vi "Generate Failure Nodes.vi"(10 "Result":T1, 11 "XML Report in":refnum<class "XML Report.lvclass">) -> (3 "XML Report out":refnum<class "XML Report.lvclass">)   [LabVIEW 2020, in "Reports.lvlib" / "XML Report.lvclass"]
uses:
  XML Report.lvclass
  Core/Result/Result.ctl
  Core/Result/Status.ctl
  Core/Result/Type.ctl
  XML Report.lvclass/XML Report.ctl
  <vilib>/Utility/miscctls.llb/LVMapReplaceAction.ctl
  <resource>/objmgr/DOMUserDefRef.rc
  Framework/Utilities/Utilities.lvlib
  Core/Result/Result.lvlib
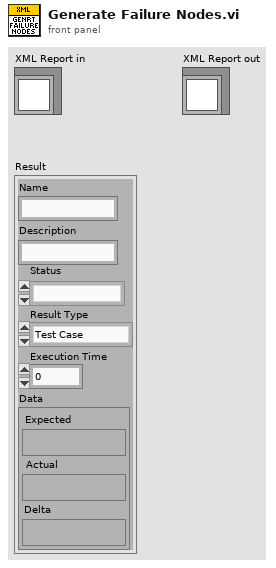
[diagram p1: front panel]
types:
  T1 = typedef "Result.lvlib/Result.ctl" = cluster{"Name":string, "Description":string, "Status":T2, "Result Type":T3, "Execution Time":dbl, "Data":cluster{"Expected":variant, "Actual":variant, "Delta":variant}}
  T2 = typedef "Result.lvlib/Status.ctl" = enum16{"", "Passed", "Failed", "Error", "Skipped", "Setup Error", "Broken", "Teardown Error"}
  T3 = typedef "Result.lvlib/Type.ctl" = enum16{"Test Case", "Test Suite", "Test Run", "Pass", "Fail", "Skip", "Pass if", "Fail if", "Pass if Error", "Fail if Error", "Pass if Equal", "Fail if Equal"}
  T4 = typedef "LVMapReplaceAction.ctl" = enum32{"Modify Entry only if found", "Add or Modify Entry", "Delete Entry"}
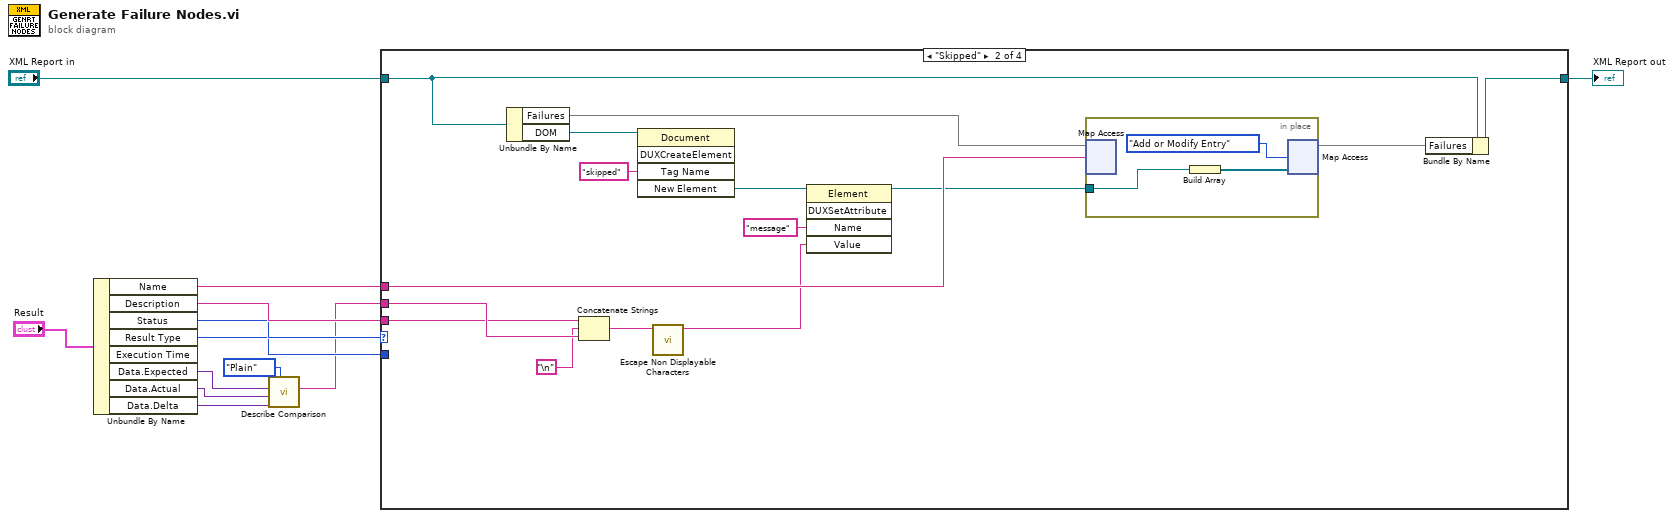
[diagram p0: block diagram]
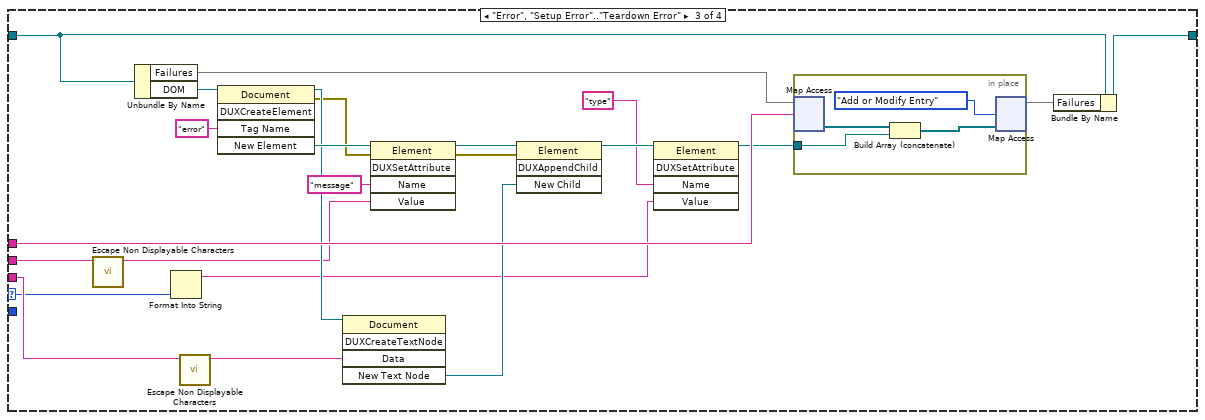
[diagram p3: hidden frame]
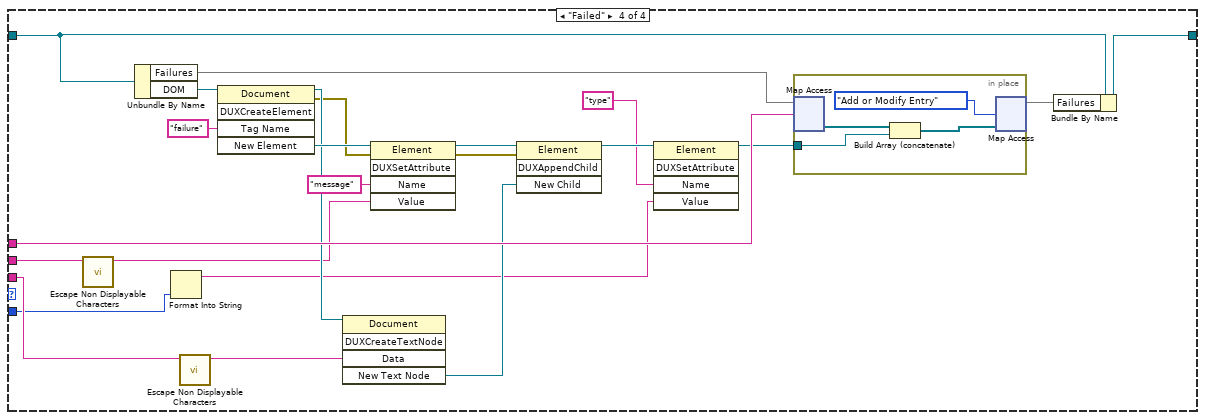
[diagram p4: hidden frame]
diagram:
  n1 = Unbundle By Name("Result") -> ("Name"=w9:string, "Description"=w8:string, "Status"=w7:T2, "Result Type"=w6:T3, "Data.Expected"=w5:variant, "Data.Actual"=w4:variant, "Data.Delta"=w3:variant)  [unwired: 1 out]
  n2 = call "Describe Comparison.vi"("Delta"=w3, "Style"=enum16{"Diff", "Plain"}."Plain", "Actual"=w4, "Expected"=w5) -> ("Description"=w2:string)  [unwired: 7 in]
  n3 = case shown="\"Skipped\"" w7 {
    selector: w7 -> [_ _ w36 _]
    tunnel: [w13 w28 w54 w81] -> w11
    tunnel: "XML Report in" -> [w13 w27 w53 w80]
    tunnel: w9 -> [_ w23 w49 w76]
    tunnel: w2 -> [_ w18 w33 w72]
    tunnel: w8 -> [_ w16 w44 w70]
    tunnel: w6 -> [_ _ _ w61]
    frame "", "Passed" {
    }
    frame "Skipped" {
      n4 = Unbundle By Name(w27) -> ("Failures"=w24:map{string, refnum<k20>[]}, "DOM"=w26:refnum<k20>)
      n5 = Concatenate Strings(w16, "\n", w18) -> (w17:string)
      n6 = invoke class="Document" method="DUXCreateElement"(reference=w26, "Tag Name"="skipped") -> ("New Element"=w22:refnum<k20>)  [unwired: 3 in, 4 out]
      n7 = call "Escape Non Displayable Characters.vi"("Raw String"=w17) -> ("Escaped String"=w14:string)  [unwired: 10 in]
      n8 = invoke class="Element" method="DUXSetAttribute"(reference=w22, "Name"="message", "Value"=w14) -> (reference out=w20:refnum<k20>)  [unwired: 2 in, 4 out]
      n9 = in-place {
        in-place-border: w20 -> [w31]
        n10 = in-place-map #1(w24, w23) -> ()  [unwired: 1 in, 2 out]
        n11 = Build Array(w31) -> (w29:refnum<k20>[])
        n12 = in-place-map #1(w29, LVMapReplaceAction."Add or Modify Entry" ("action")) -> (w21:map{string, refnum<k20>[]})  [unwired: 2 out]
      }
      n13 = Bundle By Name(cluster=w27, "Failures"=w21) -> (w28:refnum<class "XML Report.lvclass">)
    }
    frame "Error", "Setup Error".."Teardown Error" {
      n14 = call "Escape Non Displayable Characters.vi"("Raw String"=w33) -> ("Escaped String"=w32:string)  [unwired: 10 in]
      n15 = Unbundle By Name(w53) -> ("Failures"=w50:map{string, refnum<k20>[]}, "DOM"=w52:refnum<k20>)
      n16 = Format Into String(w36) -> (resulting string=w35:string)  [unwired: 3 in, 1 out]
      n17 = call "Escape Non Displayable Characters.vi"("Raw String"=w44) -> ("Escaped String"=w34:string)  [unwired: 10 in]
      n18 = invoke class="Document" method="DUXCreateElement"(reference=w52, "Tag Name"="error") -> (reference out=w45:refnum<k20>, error out=w40:errorcluster, "New Element"=w48:refnum<k20>)  [unwired: 3 in, 2 out]
      n19 = invoke class="Document" method="DUXCreateTextNode"(reference=w45, "Data"=w34) -> ("New Text Node"=w41:refnum<k20>)  [unwired: 3 in, 4 out]
      n20 = invoke class="Element" method="DUXSetAttribute"(reference=w48, error in=w40, "Name"="message", "Value"=w32) -> (reference out=w43:refnum<k20>, error out=w39:errorcluster)  [unwired: 1 in, 3 out]
      n21 = invoke class="Element" method="DUXAppendChild"(reference=w43, error in=w39, "New Child"=w41) -> (reference out=w42:refnum<k20>)  [unwired: 1 in, 3 out]
      n22 = invoke class="Element" method="DUXSetAttribute"(reference=w42, "Name"="type", "Value"=w35) -> (reference out=w38:refnum<k20>)  [unwired: 2 in, 4 out]
      n23 = in-place {
        in-place-border: w38 -> [w57]
        n24 = in-place-map #2(w50, w49) -> (w58:refnum<k20>[])  [unwired: 1 in, 1 out]
        n25 = Build Array (concatenate)(w58, w57) -> (w55:refnum<k20>[])
        n26 = in-place-map #2(w55, LVMapReplaceAction."Add or Modify Entry" ("action")) -> (w47:map{string, refnum<k20>[]})  [unwired: 2 out]
      }
      n27 = Bundle By Name(cluster=w53, "Failures"=w47) -> (w54:refnum<class "XML Report.lvclass">)
    }
    frame "Failed" {
      n28 = call "Escape Non Displayable Characters.vi"("Raw String"=w72) -> ("Escaped String"=w60:string)  [unwired: 10 in]
      n29 = Unbundle By Name(w80) -> ("Failures"=w77:map{string, refnum<k20>[]}, "DOM"=w79:refnum<k20>)
      n30 = Format Into String(w61) -> (resulting string=w62:string)  [unwired: 3 in, 1 out]
      n31 = call "Escape Non Displayable Characters.vi"("Raw String"=w70) -> ("Escaped String"=w59:string)  [unwired: 10 in]
      n32 = invoke class="Document" method="DUXCreateElement"(reference=w79, "Tag Name"="failure") -> (reference out=w71:refnum<k20>, error out=w66:errorcluster, "New Element"=w75:refnum<k20>)  [unwired: 3 in, 2 out]
      n33 = invoke class="Document" method="DUXCreateTextNode"(reference=w71, "Data"=w59) -> ("New Text Node"=w67:refnum<k20>)  [unwired: 3 in, 4 out]
      n34 = invoke class="Element" method="DUXSetAttribute"(reference=w75, error in=w66, "Name"="message", "Value"=w60) -> (reference out=w69:refnum<k20>, error out=w65:errorcluster)  [unwired: 1 in, 3 out]
      n35 = invoke class="Element" method="DUXAppendChild"(reference=w69, error in=w65, "New Child"=w67) -> (reference out=w68:refnum<k20>)  [unwired: 1 in, 3 out]
      n36 = invoke class="Element" method="DUXSetAttribute"(reference=w68, "Name"="type", "Value"=w62) -> (reference out=w64:refnum<k20>)  [unwired: 2 in, 4 out]
      n37 = in-place {
        in-place-border: w64 -> [w84]
        n38 = in-place-map #3(w77, w76) -> (w85:refnum<k20>[])  [unwired: 1 in, 1 out]
        n39 = Build Array (concatenate)(w85, w84) -> (w82:refnum<k20>[])
        n40 = in-place-map #3(w82, LVMapReplaceAction."Add or Modify Entry" ("action")) -> (w74:map{string, refnum<k20>[]})  [unwired: 2 out]
      }
      n41 = Bundle By Name(cluster=w80, "Failures"=w74) -> (w81:refnum<class "XML Report.lvclass">)
    }
  }
  "XML Report out" <- w11
